vi "95-5 Filter.vi"(1 "In":dbl, 2 "Percent":dbl) -> (0 "Out":dbl)   [LabVIEW 2015]
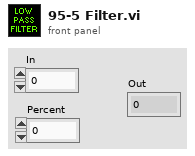
[diagram p1: front panel]
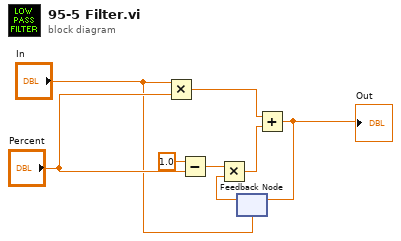
[diagram p0: block diagram]
diagram:
  n1 = Multiply(x="In", y="Percent") -> (x*y=w6:dbl)
  n2 = Subtract(x=1.0 ("y"), y="Percent") -> (x-y=w8:dbl)
  n3 = feedback #1("In") -> (w5:dbl)
  n4 = Multiply(x=w8, y=w5) -> (x*y=w7:dbl)
  n5 = Add(x=w6, y=w7) -> (x+y=w1:dbl)
  "Out" <- w1
  n6 = feedback-in #1(w1) -> ()
